vi "1D Array (Random[0,N-1]).vi"(1 "Length":u64, 4 "Dimension":u64) -> (15 "Array":u64[](array[numeric]))   [LabVIEW 2014]
panel:
  out "fails":i32
  in  "tolerance":dbl
  out "expected":dbl format="%_4f"
  out "mean":dbl format="%_4f"
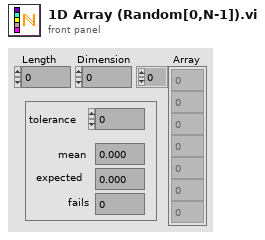
[diagram p1: front panel]
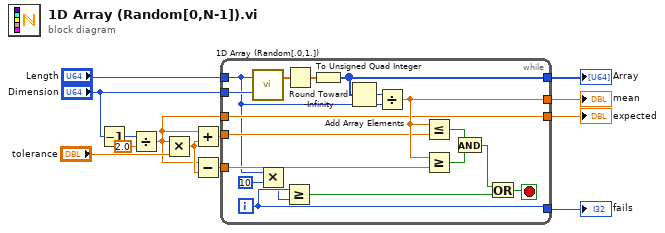
[diagram p0: block diagram]
diagram:
  n1 = Decrement(x="Dimension") -> (x-1=w8:u64)
  n2 = Divide(x=w8, y=2.0) -> (x/y=w3:dbl)
  n3 = Multiply(x=w3, y="tolerance") -> (x*y=w6:dbl)
  n4 = Add(x=w3, y=w6) -> (x+y=w5:dbl)
  n5 = Subtract(x=w3, y=w6) -> (x-y=w4:dbl)
  n6 = while {
    tunnel: [w31] -> w13
    tunnel: [w24] -> w12
    tunnel: "Length" -> [w15]
    tunnel: "Dimension" -> [w27]
    tunnel: w5 -> [w23]
    tunnel: w4 -> [w22]
    tunnel: w3 -> [w18]
    tunnel: [w18] -> w2
    tunnel: [w17] -> w1
    i -> [w17]
    stop <- w26 stop-if-true
    n7 = call "1D Array (Random[.0,1.]).vi"("Length"=w15, "Scale(1.0)"=w27) -> ("Array"=w28:dbl[])  [unwired: 17 in]
    n8 = Multiply(x=w15, y=u64 10) -> (x*y=w16:u64)
    n9 = Greater Or Equal?(x=w17, y=w16) -> (x >= y?=w25:bool)
    n10 = Round Toward -Infinity(1:w28) -> (0:w29:dbl[])
    n11 = To Unsigned Quad Integer(1:w29) -> (0:w31:u64[])
    n12 = Add Array Elements(numeric array=w31) -> (sum=w30:u64)
    n13 = Divide(x=w30, y=w15) -> (x/y=w24:dbl)
    n14 = Less Or Equal?(x=w24, y=w23) -> (x <= y?=w20:bool)
    n15 = Greater Or Equal?(x=w24, y=w22) -> (x >= y?=w21:bool)
    n16 = And(x=w20, y=w21) -> (x .and. y?=w19:bool)
    n17 = Or(x=w19, y=w25) -> (x .or. y?=w26:bool)
  }
  "Array" <- w13
  "mean" <- w12
  "expected" <- w2
  "fails" <- w1
